vi "Design Inverse Filter.vi"() -> ()   [LabVIEW 2015]
uses:
  Signal Synthesis VIs/Controls/Waveform XCtl/Waveform Enum.ctl
  Signal Synthesis VIs/Controls/Level XCtl/Level Modes.ctl
  Utility VIs/Math VIs/FFT x(t) to dB,Degrees (1D).vi
  Utility VIs/Math VIs/LinSpace (x0-dx-npts).vi
  <vilib>/Analysis/NI_AALPro.lvlib
  <vilib>/Analysis/5stat.llb/RMS (DBL).vi
  Cochlear Function Test Suite/LV Source/ABR VIs/SubVIs/ABR-Globals.vi
  Signal Synthesis VIs/Controls/Stimulus Channel (Full)/Stimulus Channel (Full).xctl
  Signal Synthesis VIs/Controls/Advanced Filter XCtl/Advanced Filter XCtl.xctl
  Signal Synthesis VIs/Controls/Level XCtl/Level XCtl.xctl
  Cochlear Function Test Suite/LV Source/ABR VIs/TypeDefs/ABR3-Masker Spec.ctl
panel:
  out "rms value":dbl format="%0.2f"
  in  "Sampling rate (Hz)":dbl
  in  "Masker":T1
  out "Max Level (compensated)":dbl
  out "Max Level":dbl caption="Max Level (uncompensated)"
  out "Noise Spectrum":cluster{"Frequency":dbl[], "Mag":dbl[]}(graph)
  in  "Stimulus Channel":T23(xcontrol)
  out "ASTF mag":cluster{"Frequency":dbl[], "Mag":dbl[]}(graph)
  in  "Calibration file":path
  out "Noise":dbl[](graph)
  in  "Design":bool
  in  "Return":bool
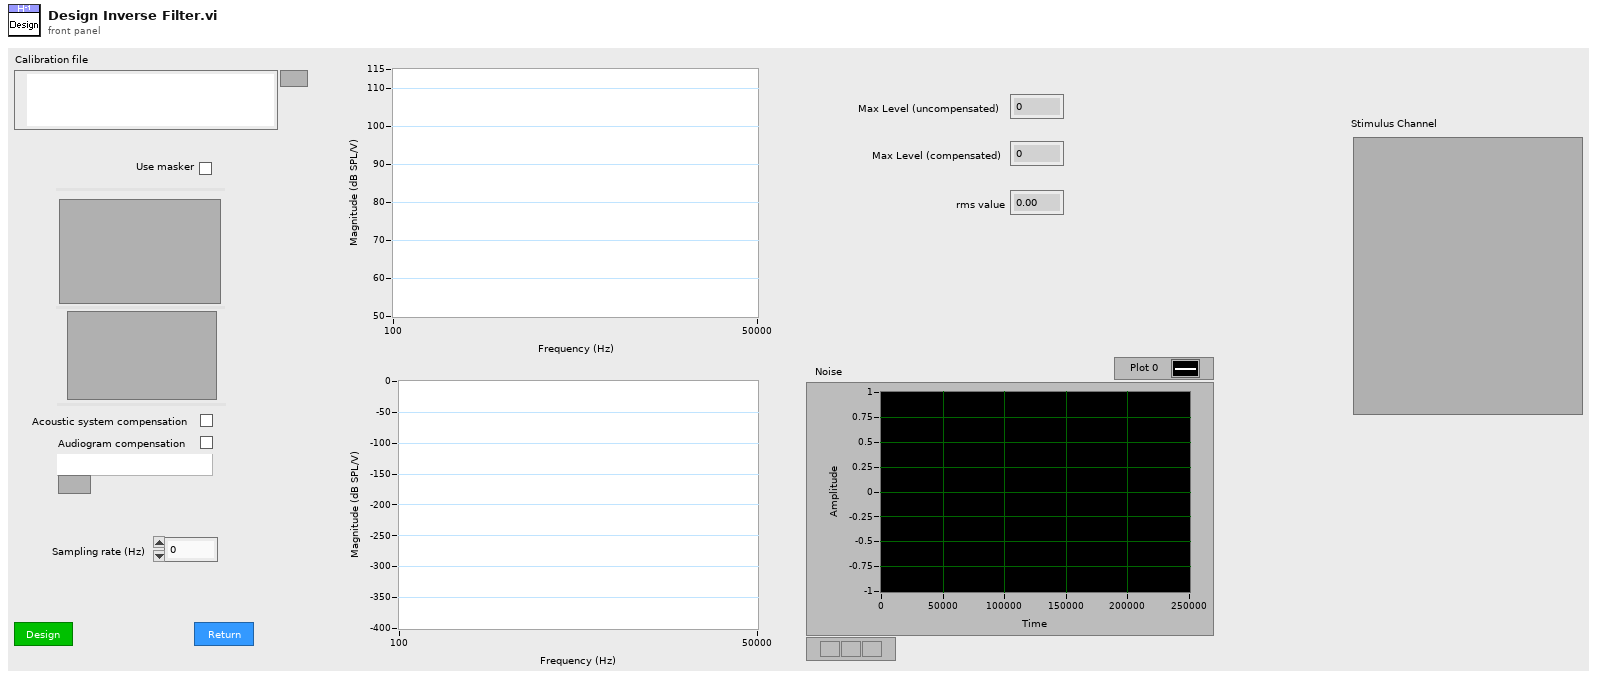
[diagram p1: front panel]
types:
  T1 = typedef "ABR3-Masker Spec.ctl" = cluster{"Filter":cluster{"Type":enum16{"Lowpass", "Highpass", "Bandpass", "Bandstop", "OFF"}, "CF (kHz)":dbl, "BW (kHz)":dbl, "Cascade":bool, "Quadrature":bool, "Scale Factor":dbl, "Stages":cluster{"IIR Filter":cluster{"filter structure":enum32{"IIR 2nd Order", "IIR 4th Order"}, "Reverse Coefficients":dbl[], "Forward Coefficients":dbl[]}, "State":dbl[]}[], "Class":enum16{"Elliptic", "Butterworth"}, "Order":i32, "BWUnits":T2}, "Use masker":bool, "Level":cluster{"Level":dbl, "Units":T3, "Max":dbl, "Multiplier":dbl, "Cal File":path, "Cal":cluster{"Freq (Hz)":dbl[], "Mag (dB SPL)":dbl[], "Phase (deg)":dbl[]}}, "Audiogram Comp":bool, "Audiogram File":path, "InvFilt":bool}
  T2 = typedef "Filter-Bandwidth Units.ctl" = enum16{"Linear", "Octaves"}
  T3 = typedef "Level Units.ctl" = enum16{"dB atten", "dB SPL", "dB re 1 Vrms", "dB V/Hz½", "mW", "dB SL"}
  T4 = typedef "Waveform XCtl.xctl/Waveform Data.ctl" = cluster{"Type":T5, "Tone":T6, "Pulse Train":T7, "Noise":T10, "File":T11, "FMSweep":T12, "Chirp Train":T13, "Complex Tone":cluster{"Params":T15, "Data":T17}}
  T5 = typedef "Waveform Enum.ctl" = enum16{"OFF", "Tone", "Noise", "Pulse Train", "File", "FM Sweep", "Chirp Train", "Complex Tone"}
  T6 = typedef "Tone Params.ctl" = cluster{"Frequency (kHz)":dbl, "Last Freq":dbl, "Last Phase":dbl}
  T7 = typedef "Pulse Train Params.ctl" = cluster{"Pulse width (us)":dbl, "Pulse rate (Hz)":dbl, "Gap (ms)":dbl, "Polarity":T8, "PT State":T9, "Asynch":bool}
  T8 = typedef "Pulse Polarity.ctl" = enum16{"POS", "NEG", "POS-NEG", "NEG-POS"}
  T9 = typedef "PT-Continuous State.ctl" = cluster{"Template":dbl[], "Nperiod":i32, "Index":i32, "Pulse Rate (Hz)":dbl, "Phase (cycles)":dbl, "Noff":i32}
  T10 = typedef "Noise Params.ctl" = cluster{"InvFilt":bool, "Noise":dbl[], "CurPt":i32, "Aweight":bool}
  T11 = typedef "StimFile-Params.ctl" = cluster{"Filename":path, "Signal":dbl[], "Channel":i32}
  T12 = typedef "FM Sweep Params.ctl" = cluster{"Rate (oct/s)":dbl, "Fmin (Hz)":dbl, "Fmax (Hz)":dbl, "Ramp (ms)":dbl, "Linear":bool}
  T13 = typedef "Chirp Train.ctl" = cluster{"Params":T14, "Data":cluster{"WF":dbl[]}}
  T14 = typedef "Chirp Train Params.ctl" = cluster{"Fmin (kHz)":dbl, "Fmax (kHz)":dbl, "Compensate":bool, "Duration (ms)":dbl}
  T15 = typedef "CT-Params.ctl" = cluster{"F0 (Hz)":dbl, "Band":cluster{"Flow (Hz)":dbl, "Fhigh (Hz)":dbl}, "Phase":T16, "Min F0 (Hz)":dbl, "Max F0 (Hz)":dbl, "ContinRandPhase":bool, "Max peak factor":dbl, "Max mod depth":dbl}
  T16 = typedef "CT-Phase Enum.ctl" = enum16{"Cosine", "Random", "Alternating"}
  T17 = typedef "CT-Runtime Data.ctl" = cluster{"Ncomp":i32, "MinHarm":i32, "Phase":dbl[], "Amplitude":dbl[], "Npts/frame":i32, "Last F0":dbl, "Fmin":dbl, "Fmax":dbl, "Lslope":dbl, "randphase":bool}
  T18 = typedef "Advanced Filter XCtl.xctl/Filter Data.ctl" = cluster{"Type":enum16{"Lowpass", "Highpass", "Bandpass", "Bandstop", "OFF"}, "CF (kHz)":dbl, "BW (kHz)":dbl, "Cascade":bool, "Quadrature":bool, "Scale Factor":dbl, "Stages":cluster{"IIR Filter":cluster{"filter structure":enum32{"IIR 2nd Order", "IIR 4th Order"}, "Reverse Coefficients":dbl[], "Forward Coefficients":dbl[]}, "State":dbl[]}[], "Class":enum16{"Elliptic", "Butterworth"}, "Order":i32, "BWUnits":T2}
  T19 = typedef "Burst Control.xctl/Burst Data.ctl" = cluster{"Active":bool, "Delay (ms)":dbl, "Duration (ms)":dbl, "Ramp (ms)":dbl, "Rate (Hz)":dbl, "Trepeat (ms)":dbl, "Repeat":bool}
  T20 = typedef "Level XCtl.xctl/Level Data.ctl" = cluster{"Level":dbl, "Units":T3, "Max":dbl, "Multiplier":dbl, "Cal File":path, "Cal":cluster{"Freq (Hz)":dbl[], "Mag (dB SPL)":dbl[], "Phase (deg)":dbl[]}}
  T21 = typedef "Advanced Stimulus Options.xctl/Advanced Stimulus Options.ctl" = cluster{"Rep Mask":string, "AltPol":bool, "Var":string, "Expr":string}
  T22 = typedef "SAM Params.ctl" = cluster{"Active":bool, "Frequency (Hz)":dbl, "Depth":dbl, "Init Phase (cycles)":dbl, "phase (degrees)":dbl, "Asynch":bool}
  T23 = cluster{"Waveform":T4, "Filter":T18, "Burst":T19, "Level":T20, "Name":string, "Advanced":T21, "SAM":T22}
  T24 = typedef "Level Modes.ctl" = enum16{"dB atten", "dB SPL", "dB re 1 Vrms"}
  T25 = enum16{"Lowpass", "Highpass", "Bandpass", "Bandstop", "OFF"}
  T26 = typedef "Stimulus Channel (Full).xctl/Full Stimulus Channel Data.ctl" = cluster{"Waveform":T4, "Filter":T18, "Burst":T19, "Level":T20, "Name":string, "Advanced":T21, "SAM":T22}
  T27 = cluster{"Array":dbl[], "+Freq. Mag of FFT (dB rms)":dbl[]}
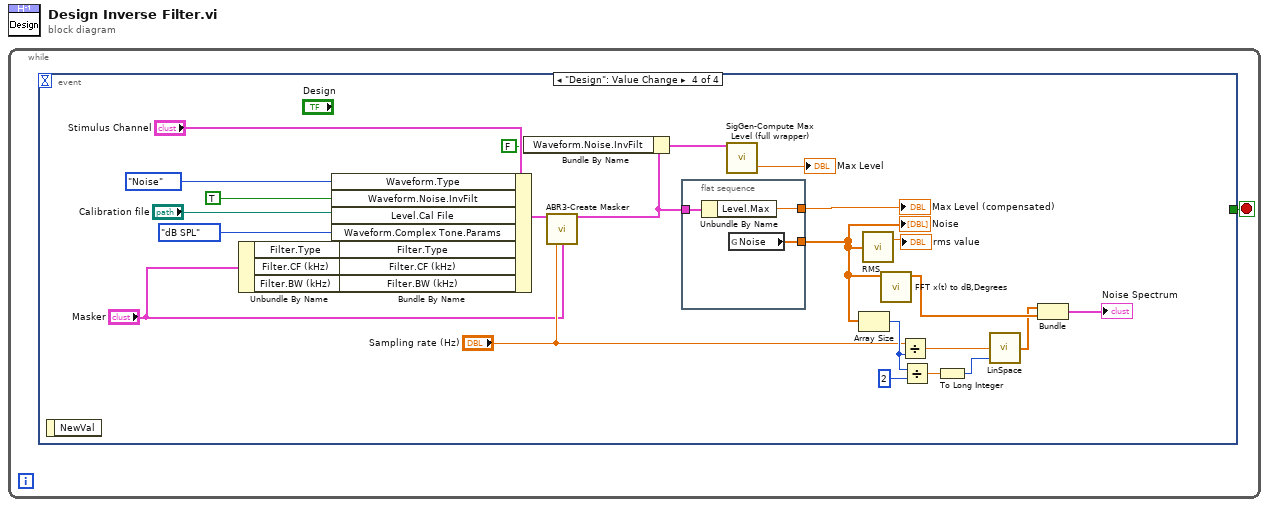
[diagram p0: block diagram]
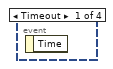
[diagram p2: hidden frame]
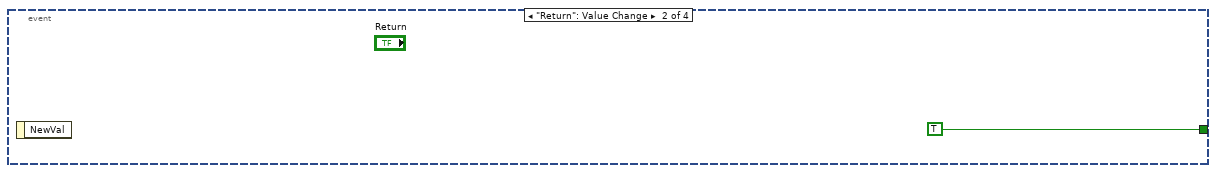
[diagram p3: hidden frame]
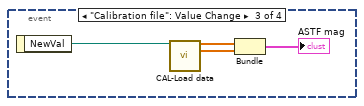
[diagram p4: hidden frame]
diagram:
  n1 = while {
    stop <- w1 stop-if-true
    n2 = event shown="[3] \"Design\": Value Change" {
      selector: _ -> [_ _ _ _]
      dyn-events: _ -> [_ _ _ _]
      timeout: _ -> [_ _ _ _]
      tunnel: [_ TRUE ("NewVal") _ _] -> w1
      event Timeout {
        n3 = event-data() -> ()  [unwired: 1 in, 1 out]
      }
      event "Return": Value Change {
        n4 = event-data() -> ()  [unwired: 1 in, 1 out]
      }
      event "Calibration file": Value Change {
        n5 = event-data() -> ("NewVal"=w6:path)  [unwired: 1 in]
        n6 = call "CAL-Load data.vi"("user path"=w6) -> ("Frequency (Hz)"=w5:dbl[], "Mag"=w4:dbl[])  [unwired: 7 in, 6 out]
        n7 = Bundle("Frequency (Hz)"=w5, "Mag"=w4) -> (→"ASTF mag":cluster{"Frequency (Hz)":dbl[], "Mag":dbl[]})  [unwired: 1 in]
      }
      event "Design": Value Change {
        n8 = event-data() -> ()  [unwired: 1 in, 1 out]
        n9 = Unbundle By Name("Masker") -> ("Filter.Type"=w11:T25, "Filter.CF (kHz)"=w10:dbl, "Filter.BW (kHz)"=w9:dbl)
        n10 = Bundle By Name(cluster="Stimulus Channel", "Waveform.Type"=Waveform_Enum."Noise", "Waveform.Noise.InvFilt"=TRUE, "Level.Cal File"="Calibration file", "Waveform.Complex Tone.Params"=Level_Modes."dB SPL" ("Level.Mode"), "Filter.Type"=w11, "Filter.CF (kHz)"=w10, "Filter.BW (kHz)"=w9) -> (w16:T23)
        n11 = call "ABR3-Create Masker.vi"("StimChan"=w16, "Sampling rate (Hz)"="Sampling rate (Hz)", "Masker"="Masker") -> ("Stimulus Channel out"=w15:T26)  [unwired: 11 in, 1 out]
        n12 = Bundle By Name(cluster=w15, "Waveform.Noise.InvFilt"=FALSE) -> (w22:T26)
        n13 = flat-sequence {
          tunnel: w15 -> [w35]
          tunnel: [w34] -> w14
          tunnel: [w33] -> w7
          frame #0 {
            n14 = Unbundle By Name(w35) -> ("Level.Max"=w34:dbl)
            n15 = global read "ABR-Globals.vi" "Noise"() -> (w33:dbl[])
          }
        }
        n16 = call "SigGen-Compute Max Level (full wrapper).vi"("Stimulus Channel"=w22) -> ("Max Level"=→"Max Level":dbl)  [unwired: 12 in, 2 out]
        n17 = Array Size(array=w7) -> (size(s)=w20:i32)
        n18 = call-poly <vilib>:"RMS.vi"("X"=w7) -> ("rms value"=→"rms value":dbl)  [unwired: 1 out]
        n19 = call-poly "FFT x(t) to dB,Degrees.vi"("X"=w7) -> ("+Freq. Mag of FFT (dB rms)"=w27:dbl[])  [unwired: 8 in, 2 out]
        n20 = Divide(x="Sampling rate (Hz)", y=w20) -> (x/y=w28:dbl)
        n21 = Divide(x=w20, y=2) -> (x/y=w18:dbl)
        n22 = To Long Integer(number=w18) -> (32bit integer=w17:i32)
        n23 = call-poly "LinSpace.vi"("npts"=w17, "dx"=w28) -> ("Array"=w26:dbl[])  [unwired: 2 in, 1 out]
        n24 = Bundle("Array"=w26, "+Freq. Mag of FFT (dB rms)"=w27) -> (→"Noise Spectrum":T27)  [unwired: 1 in]
        "Noise" <- w7
        "Max Level (compensated)" <- w14
      }
    }
  }
